vi "Channel Names FGV.vi"(6 "type":enum16{"TC", "ACC", "SG"}(ring), 7 "Config":T1={"AO config"=[], "AI config"=[], "DI config"=[], "DO config"=[], "TC config"=[], "ACC config"=[], "SG config"=[], "Strain Gauge Settings"={"poisson ratio"=0.3, "nominal gage resistance"=120.0, "gage factor"=2.08}, "bridge information"={"strain configuration"=10271, "lead wire resistance"=1.7, "initial bridge voltage"=0.0, "voltage excitation source"=10200, "voltage excitation value"=3.3}, "Sample Rate"={"AI Sample Rate"=0.0, "AO Sample Rate"=0.0, "DI Sample Rate"=0.0, "TC Sample Rate"=0.0, "DO Sample Rate"=0.0, "SG Sample Rate"=0.0, "ACC Sample Rate"=0.0}} {"bridge information"."initial bridge voltage" format="%0.2f"; "bridge information"."voltage excitation source" items=["Internal"=10200, "External"=10167, "None"=10230]; "bridge information"."voltage excitation value" format="%0.2f"; "bridge information"."lead wire resistance" format="%0.2f"; "bridge information"."strain configuration" items=["Full Bridge I"=10183, "Full Bridge II"=10184, "Full Bridge III"=10185, "Half Bridge I"=10188, "Half Bridge II"=10189, "Quarter Bridge I"=10271, "Quarter Bridge II"=10272]; "ACC config"."Terminal configuration" items=["default"=-1, "RSE"=10083, "NRSE"=10078, "Differential"=10106, "Pseudodifferential"=12529]; "ACC config"."Sensitivity units" items=["mVolts/g"=12509, "Volts/g"=12510]; "TC config"."type" items=["J"=10072, "K"=10073, "N"=10077, "R"=10082, "S"=10085, "T"=10086, "B"=10047, "E"=10055]; "TC config"."units" items=["Deg C", "Deg F", "Kelvins", "Deg R", "From Custom Scale"]}, 8 "t":bool, 9 "names":string[](array[string]), 10 "DAQ ref":T2, 11 "Channel names 2":T3) -> ()   [LabVIEW 2022 SP3]
uses:
  Controls/Config.ctl
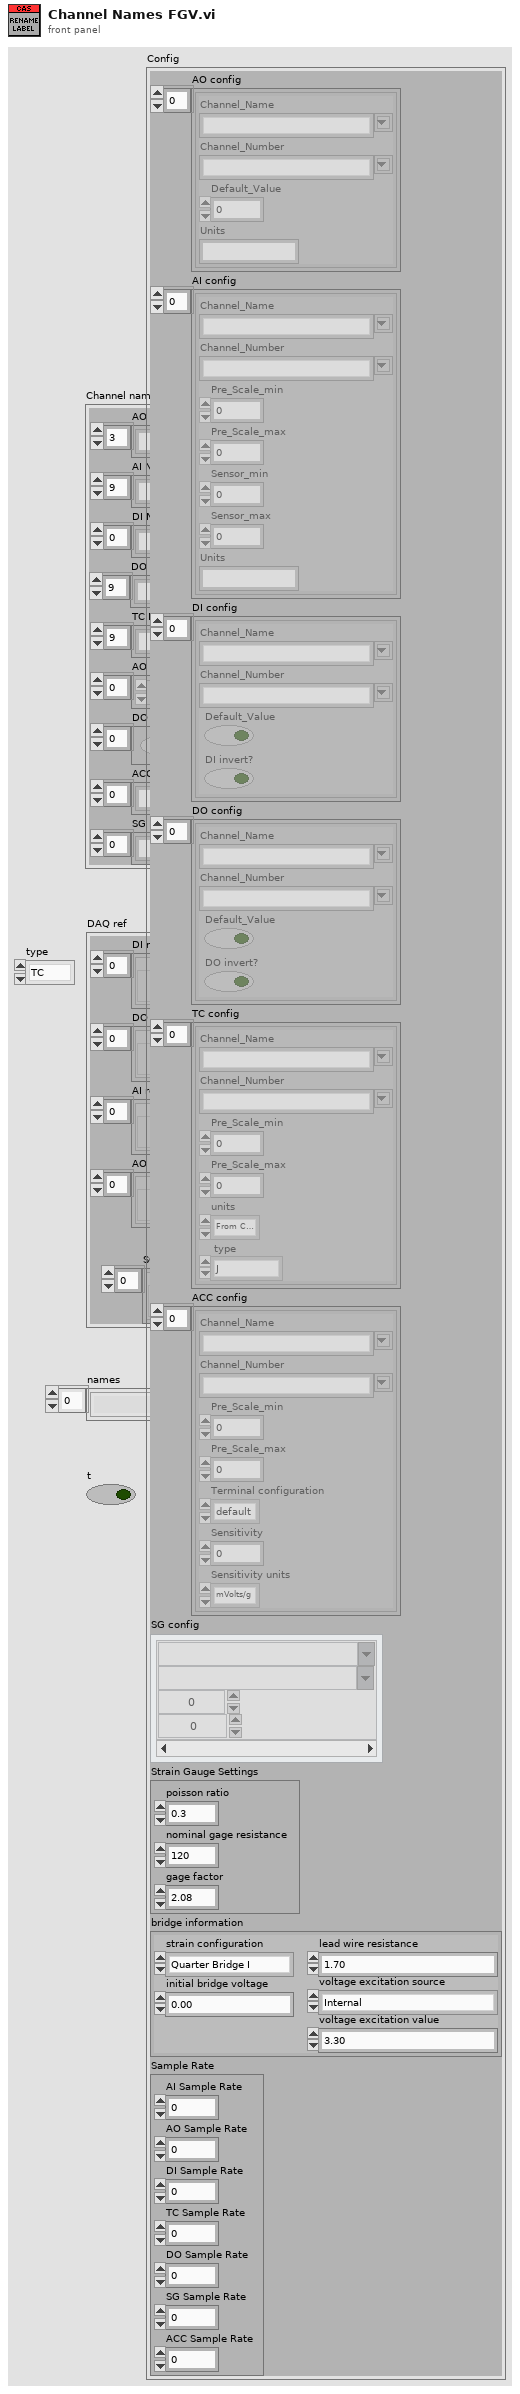
[diagram p1: front panel]
types:
  T1 = typedef "Config.ctl" = cluster{"AO config":cluster{"Channel_Name":string, "Channel_Number":string, "Default_Value":dbl, "Units":string}[], "AI config":cluster{"Channel_Name":string, "Channel_Number":string, "Pre_Scale_min":dbl, "Pre_Scale_max":dbl, "Sensor_min":dbl, "Sensor_max":dbl, "Units":string}[], "DI config":cluster{"Channel_Name":string, "Channel_Number":string, "Default_Value":bool, "DI invert?":bool}[], "DO config":cluster{"Channel_Name":string, "Channel_Number":string, "Default_Value":bool, "DO invert?":bool}[], "TC config":cluster{"Channel_Name":string, "Channel_Number":string, "Pre_Scale_min":dbl, "Pre_Scale_max":dbl, "units":i32, " type":i32}[], "ACC config":cluster{"Channel_Name":string, "Channel_Number":string, "Pre_Scale_min":dbl, "Pre_Scale_max":dbl, "Terminal configuration":i32, "Sensitivity":dbl, "Sensitivity units":i32}[], "SG config":cluster{"Channel_Name":string, "Channel_Number":string, "Pre_Scale_min":dbl, "Pre_Scale_max":dbl}[], "Strain Gauge Settings":cluster{"poisson ratio":dbl, "nominal gage resistance":dbl, "gage factor":dbl}, "bridge information":cluster{"strain configuration":i32, "lead wire resistance":dbl, "initial bridge voltage":dbl, "voltage excitation source":i32, "voltage excitation value":dbl}, "Sample Rate":cluster{"AI Sample Rate":dbl, "AO Sample Rate":dbl, "DI Sample Rate":dbl, "TC Sample Rate":dbl, "DO Sample Rate":dbl, "SG Sample Rate":dbl, "ACC Sample Rate":dbl}}
  T2 = cluster{"DI ref":refnum<vi>[], "DO ref":refnum<vi>[], "AI ref":refnum<vi>[], "AO ref":refnum<vi>[], "SG,TC,ACC":refnum<vi>[]}
  T3 = cluster{"AO Names":string[], "AI Names":string[], "DI Names":string[], "DO Names":string[], "TC Names":string[], "AO Default":dbl[], "DO Default":bool[], "ACC Names":string[], "SG Names":string[]}
  T4 = cluster{"Channel_Name":string, "Channel_Number":string, "Pre_Scale_min":dbl, "Pre_Scale_max":dbl, "Sensor_min":dbl, "Sensor_max":dbl, "Units":string}[]
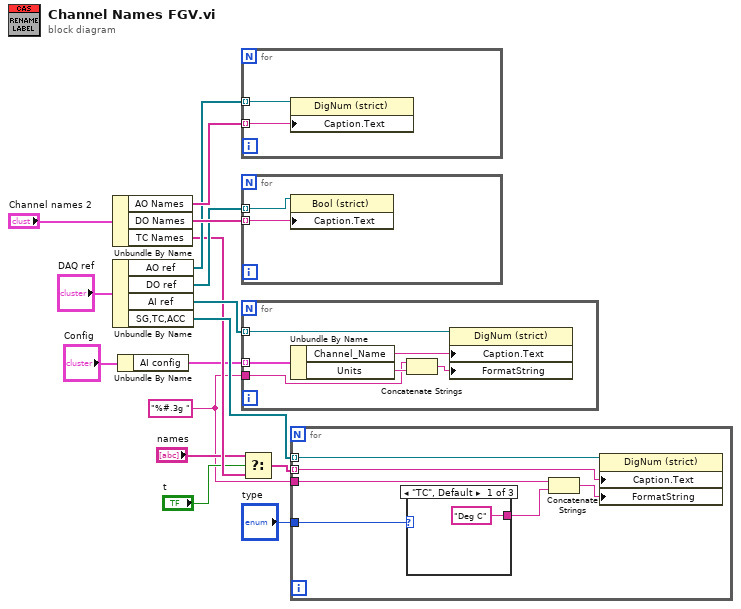
[diagram p0: block diagram]
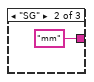
[diagram p2: hidden frame]
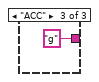
[diagram p3: hidden frame]
diagram:
  w2 = "%#.3g " ("Format String")
  n1 = Unbundle By Name("Channel names 2") -> ("AO Names"=w12:string[], "DO Names"=w15:string[], "TC Names"=w7:string[])
  n2 = Unbundle By Name("DAQ ref") -> ("AO ref"=w11:refnum<vi>[], "DO ref"=w13:refnum<vi>[], "AI ref"=w10:refnum<vi>[], "SG,TC,ACC"=w9:refnum<vi>[])
  n3 = Unbundle By Name("Config") -> ("AI config"=w4:T4)
  n4 = for {
    tunnel: w12 -> [w17] mode=indexing
    tunnel: w11 -> [w18] mode=indexing
    n5 = property class="DigNum (strict)"(reference=w18, "Caption.Text"=w17) -> ()  [unwired: 1 in, 2 out]
  }
  n6 = for {
    tunnel: w15 -> [w19] mode=indexing
    tunnel: w13 -> [w20] mode=indexing
    n7 = property class="Bool (strict)"(reference=w20, "Caption.Text"=w19) -> ()  [unwired: 1 in, 2 out]
  }
  n8 = for {
    tunnel: w10 -> [w26] mode=indexing
    tunnel: w4 -> [w25] mode=indexing
    tunnel: w2 -> [w23]
    n9 = Unbundle By Name(w25) -> ("Channel_Name"=w21:string, "Units"=w24:string)
    n10 = Concatenate Strings(w23, w24) -> (w22:string)
    n11 = property class="DigNum (strict)"(reference=w26, "Caption.Text"=w21, "FormatString"=w22) -> ()  [unwired: 1 in, 2 out]
  }
  n12 = Select(t="names", s="t", f=w7) -> (s? t:f=w8:string[])
  n13 = for {
    tunnel: w8 -> [w31] mode=indexing
    tunnel: w9 -> [w32] mode=indexing
    tunnel: w2 -> [w29]
    tunnel: "type" -> [w27]
    n14 = case shown="\"TC\", Default" w27 {
      tunnel: ["Deg C" ("string") "mm" ("string") "g" ("string")] -> w30
      frame "TC", Default {
      }
      frame "SG" {
      }
      frame "ACC" {
      }
    }
    n15 = Concatenate Strings(w29, w30) -> (w28:string)
    n16 = property class="DigNum (strict)"(reference=w32, "Caption.Text"=w31, "FormatString"=w28) -> ()  [unwired: 1 in, 2 out]
  }
